vi "test-SwerveModuleState.vi"(8 "error in (no error)":errorcluster) -> (0 "error out":errorcluster, 3 "ALL TESTS PASSED":bool)   [LabVIEW 2019]
uses:
  <vilib>/Rock Robotics/WPI/ThirdParty/JAS_Junk/TrajLib/TypeDef/SWERVE_DRIVE_MODULE_STATE.ctl
  <vilib>/Rock Robotics/WPI/ThirdParty/JAS_Junk/TrajLib/TypeDef/ROTATION2D.ctl
  <vilib>/Rock Robotics/WPI/ThirdParty/JAS_Junk/TrajLib/Rotation2d_Minus.vi
  <vilib>/Rock Robotics/WPI/ThirdParty/JAS_Junk/TrajLib/Rotation2d_GetRadians.vi
  <vilib>/Rock Robotics/WPI/ThirdParty/JAS_Junk/TrajLib/Rotation2d_RotateBy.vi
  <vilib>/Rock Robotics/WPI/ThirdParty/JAS_Junk/TrajLib/Rotation2d_UnaryMinus.vi
  <vilib>/Rock Robotics/WPI/ThirdParty/JAS_Junk/TrajLib/Rotation2d_CreateXY.vi
  <vilib>/Rock Robotics/WPI/ThirdParty/JAS_Junk/TrajLib/Util_CalcDist.vi
  <vilib>/Rock Robotics/WPI/ThirdParty/JAS_Junk/TrajLib/Trajectory_Library.lvlib
panel:
  out "Test 4":bool
  out "Test 3":bool
  out "Test 1B":bool
  out "T1B":T1={"Speed"=0.0, "Angle"={"VALUE"=0.0, "COS"=1.0, "SIN"=0.0}} {"Angle"."SIN" format="%13.4f"; "Angle"."COS" format="%13.4f"; "Angle"."VALUE" format="%13.4f"}
  out "Test 1A":bool
  out "T1A":T1={"Speed"=0.0, "Angle"={"VALUE"=0.0, "COS"=1.0, "SIN"=0.0}} {"Angle"."SIN" format="%13.4f"; "Angle"."COS" format="%13.4f"; "Angle"."VALUE" format="%13.4f"}
  out "Test 0B":bool
  out "T0B":T1={"Speed"=0.0, "Angle"={"VALUE"=0.0, "COS"=1.0, "SIN"=0.0}} {"Angle"."SIN" format="%13.4f"; "Angle"."COS" format="%13.4f"; "Angle"."VALUE" format="%13.4f"}
  out "Test 0A":bool
  out "T91 Ang = reversed":T1={"Speed"=0.0, "Angle"={"VALUE"=0.0, "COS"=1.0, "SIN"=0.0}} {"Angle"."SIN" format="%13.4f"; "Angle"."COS" format="%13.4f"; "Angle"."VALUE" format="%13.4f"}
  out "T90  Ang = small":T1={"Speed"=0.0, "Angle"={"VALUE"=0.0, "COS"=1.0, "SIN"=0.0}} {"Angle"."SIN" format="%13.4f"; "Angle"."COS" format="%13.4f"; "Angle"."VALUE" format="%13.4f"}
  out "T3":T1={"Speed"=0.0, "Angle"={"VALUE"=0.0, "COS"=1.0, "SIN"=0.0}} {"Angle"."SIN" format="%13.4f"; "Angle"."COS" format="%13.4f"; "Angle"."VALUE" format="%13.4f"}
  out "T2":T1={"Speed"=0.0, "Angle"={"VALUE"=0.0, "COS"=1.0, "SIN"=0.0}} {"Angle"."SIN" format="%13.4f"; "Angle"."COS" format="%13.4f"; "Angle"."VALUE" format="%13.4f"}
  out "T1":i32
  out "T0A":T1={"Speed"=0.0, "Angle"={"VALUE"=0.0, "COS"=1.0, "SIN"=0.0}} {"Angle"."SIN" format="%13.4f"; "Angle"."COS" format="%13.4f"; "Angle"."VALUE" format="%13.4f"}
  # "SwerveModuleState Test"
  # "THESE ARE OLD TESTS..."
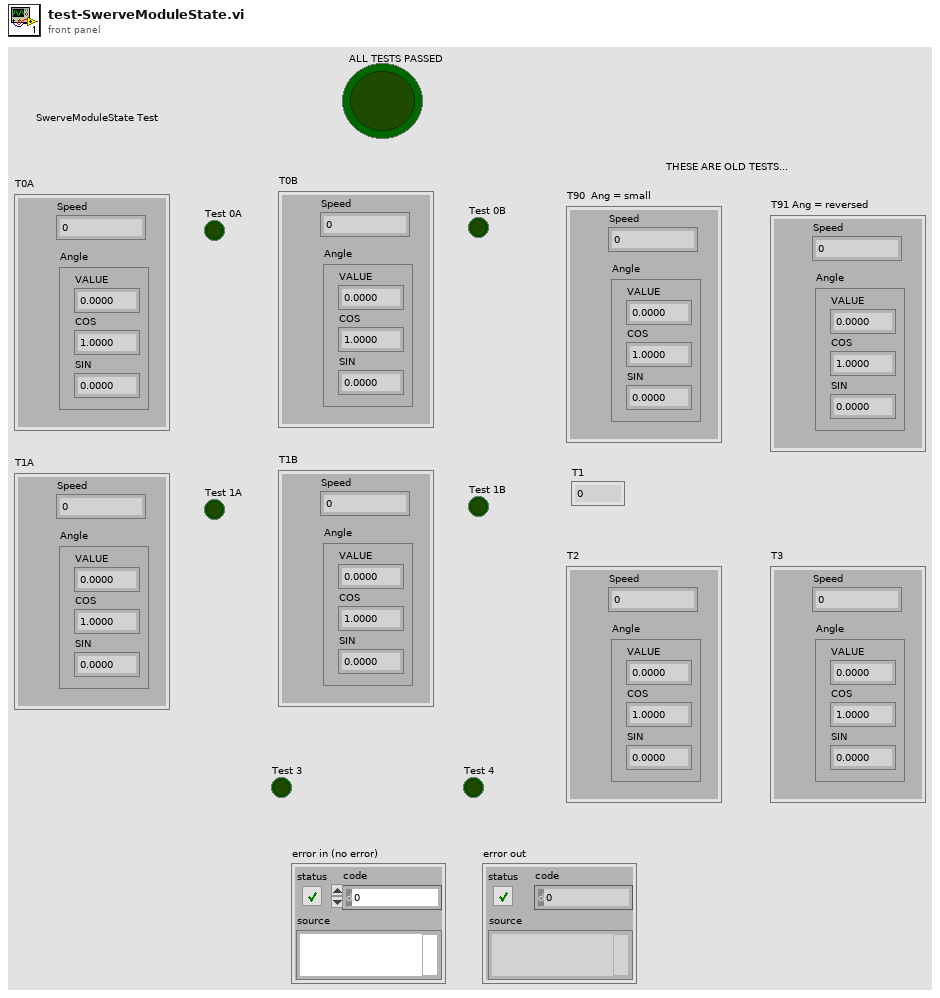
[diagram p1: front panel]
types:
  T1 = typedef "Trajectory_Library.lvlib/SWERVE_DRIVE_MODULE_STATE.ctl" = cluster{"Speed":dbl, "Angle":T2}
  T2 = typedef "Trajectory_Library.lvlib/ROTATION2D.ctl" = cluster{"VALUE":dbl, "COS":dbl, "SIN":dbl}
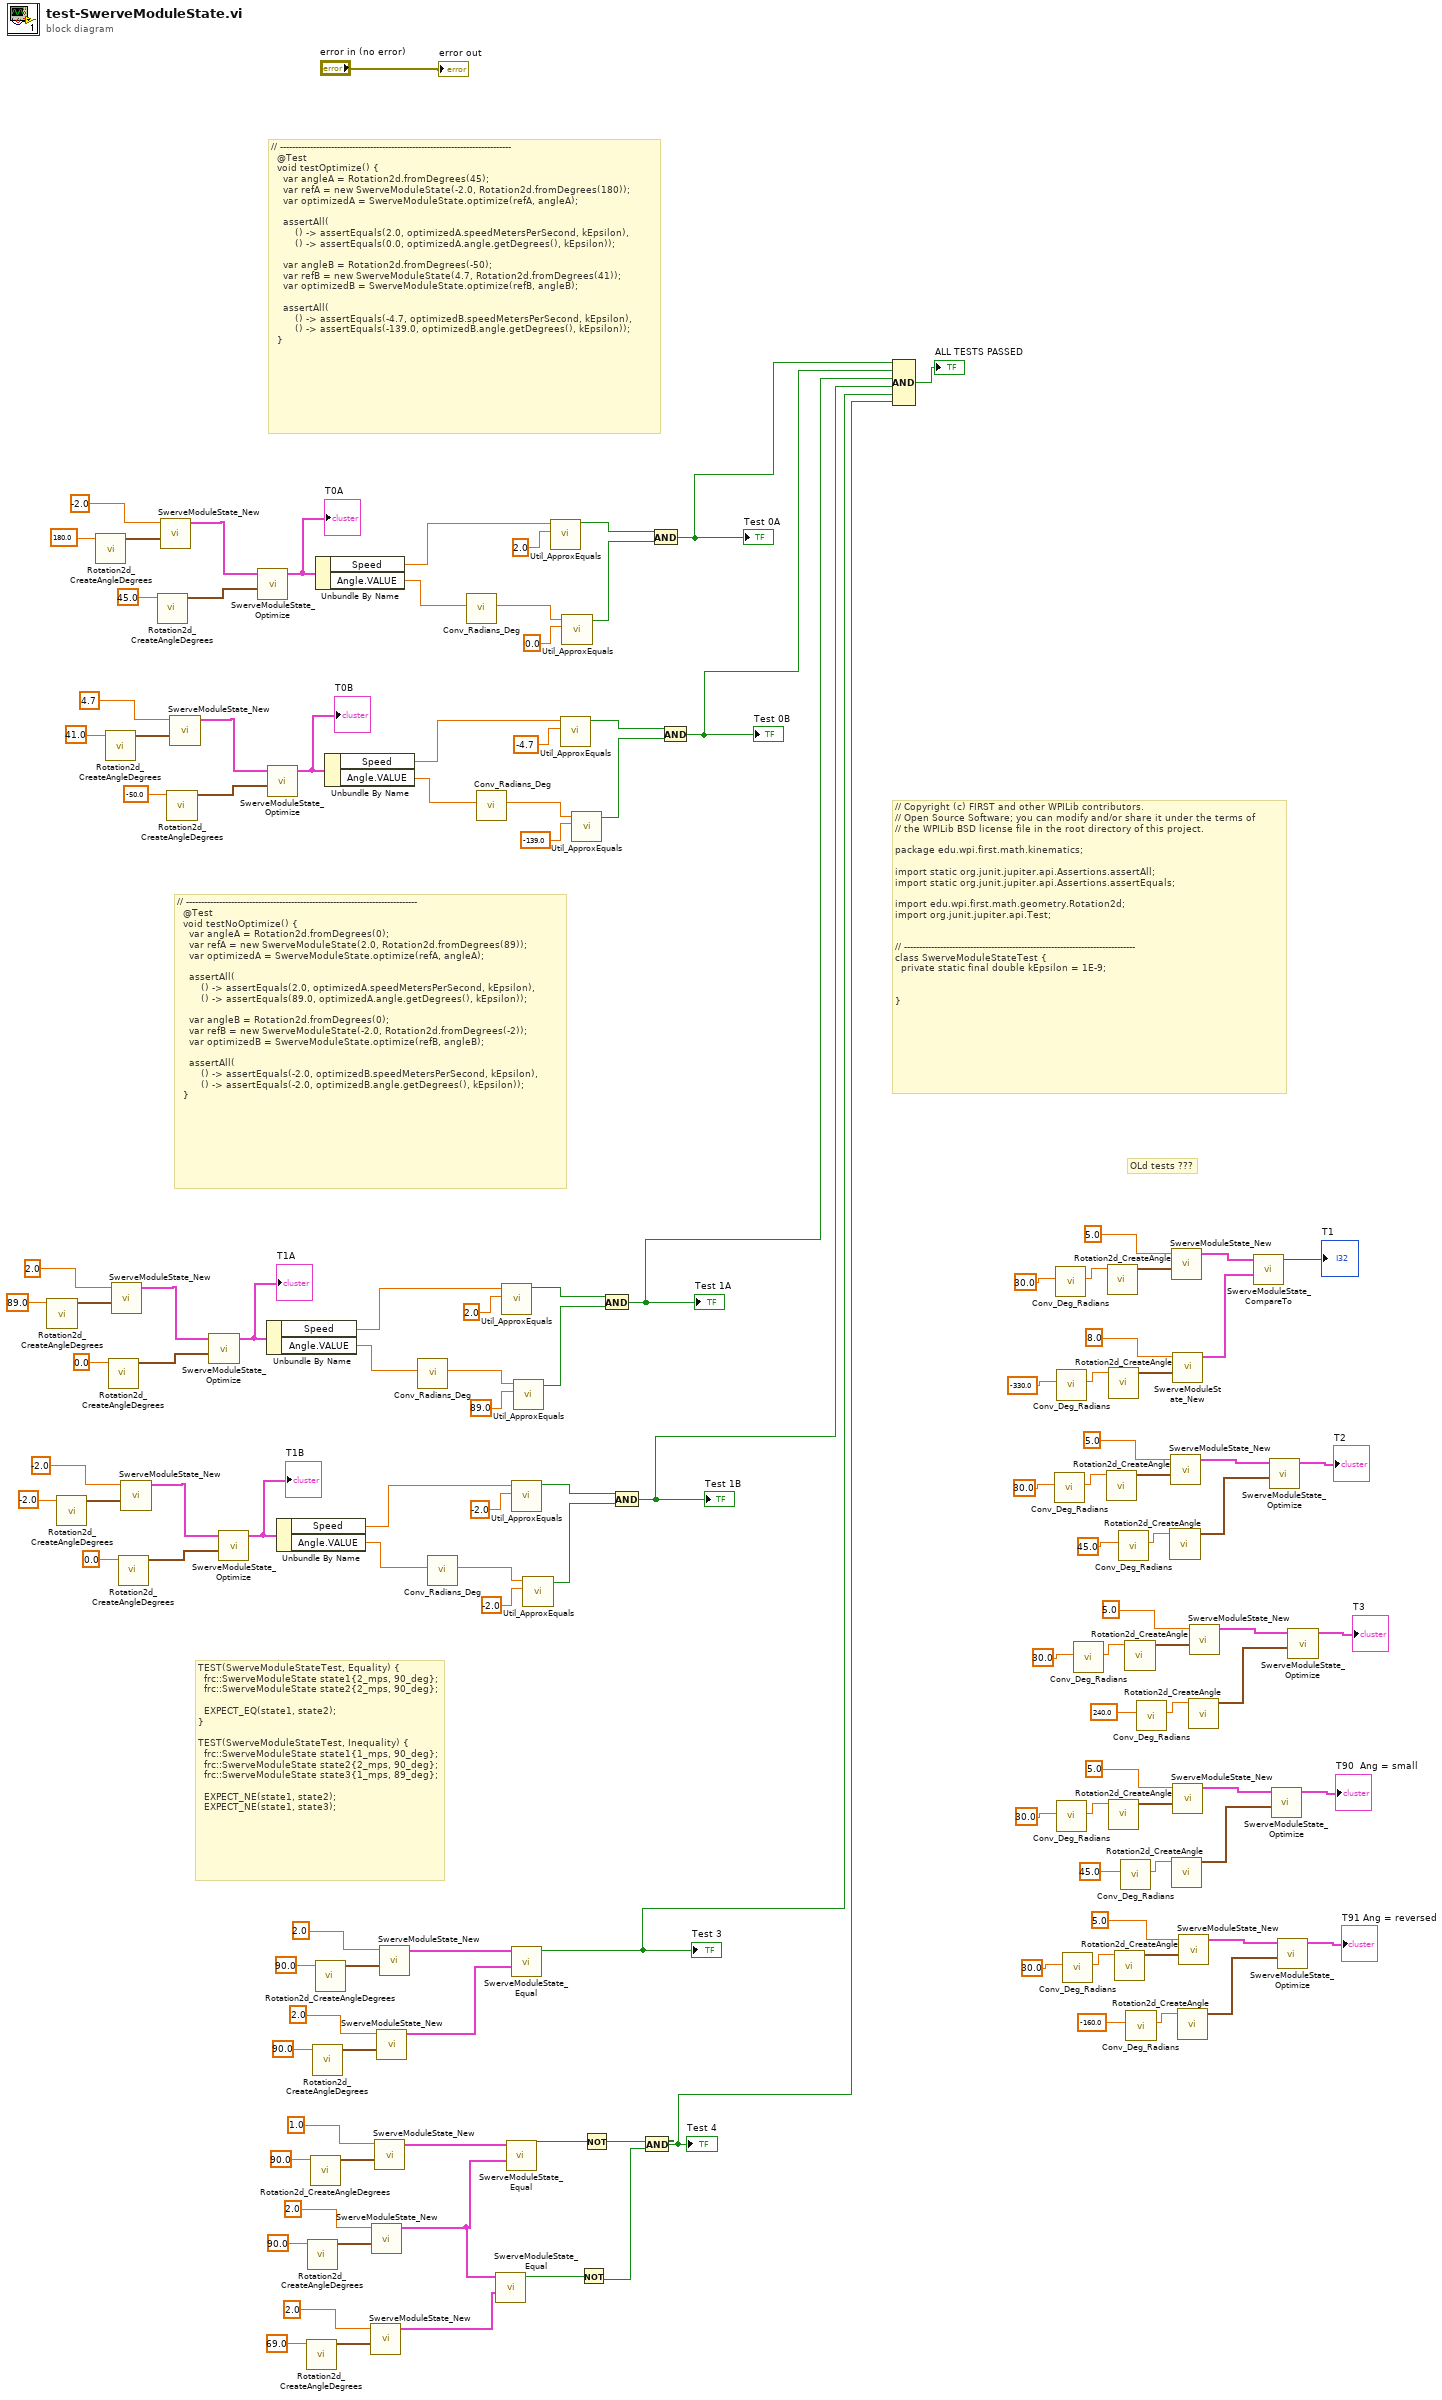
[diagram p0: block diagram]
diagram:
  # "TEST(SwerveModuleStateTest, Equality) {\n  frc::SwerveModuleState state1{2_mps, 90_deg};\n  frc::SwerveModuleState state2{2_mps, 90_deg};\n\n  EXPECT_EQ(state1, state2);\n}\n\nTEST(SwerveModuleStateTest, Inequality) {\n  frc::SwerveModuleState state1{1_mps, 90_deg};\n  frc::SwerveModuleState state2{2_mps, 90_deg};\n  frc::SwerveModuleState state3{1_mps, 89_deg};\n\n  EXPECT_NE(state1, state2);\n  EXPECT_NE(state1, state3);"
  # "OLd tests ???"
  # "// -----------------------------------------------------------------------------\n  @Test\n  void testNoOptimize() {\n    var angleA = Rotation2d.fromDegrees(0);\n    var refA = new SwerveModuleState(2.0, Rotation2d.fromDegrees(89));\n    var optimizedA = SwerveModuleState.optimize(refA, angleA);\n\n    assertAll(\n        () -> assertEquals(2.0, optimizedA.speedMetersPerSecond, kEpsilon),\n        () -> assertEquals(89.0, optimizedA.angle.getDegrees(), kEpsilon));\n\n    var angleB = Rotation2d.fromDegrees(0);\n    var refB = new SwerveModuleState(-2.0, Rotation2d.fromDegrees(-2));\n    var optimizedB = SwerveModuleState.optimize(refB, angleB);\n\n    assertAll(\n        () -> assertEquals(-2.0, optimizedB.speedMetersPerSecond, kEpsilon),\n        () -> assertEquals(-2.0, optimizedB.angle.getDegrees(), kEpsilon));\n  }"
  # "// -----------------------------------------------------------------------------\n  @Test\n  void testOptimize() {\n    var angleA = Rotation2d.fromDegrees(45);\n    var refA = new SwerveModuleState(-2.0, Rotation2d.fromDegrees(180));\n    var optimizedA = SwerveModuleState.optimize(refA, angleA);\n\n    assertAll(\n        () -> assertEquals(2.0, optimizedA.speedMetersPerSecond, kEpsilon),\n        () -> assertEquals(0.0, optimizedA.angle.getDegrees(), kEpsilon));\n\n    var angleB = Rotation2d.fromDegrees(-50);\n    var refB = new SwerveModuleState(4.7, Rotation2d.fromDegrees(41));\n    var optimizedB = SwerveModuleState.optimize(refB, angleB);\n\n    assertAll(\n        () -> assertEquals(-4.7, optimizedB.speedMetersPerSecond, kEpsilon),\n        () -> assertEquals(-139.0, optimizedB.angle.getDegrees(), kEpsilon));\n  }"
  # "// Copyright (c) FIRST and other WPILib contributors.\n// Open Source Software; you can modify and/or share it under the terms of\n// the WPILib BSD license file in the root directory of this project.\n\npackage edu.wpi.first.math.kinematics;\n\nimport static org.junit.jupiter.api.Assertions.assertAll;\nimport static org.junit.jupiter.api.Assertions.assertEquals;\n\nimport edu.wpi.first.math.geometry.Rotation2d;\nimport org.junit.jupiter.api.Test;\n\n\n// -----------------------------------------------------------------------------\nclass SwerveModuleStateTest {\n  private static final double kEpsilon = 1E-9;\n\n\n}"
  n1 = call <vilib>:"Rotation2d_CreateAngleDegrees.vi"("Angle_Degrees"=89.0 ("y")) -> ("ROTATION"=w56:T2)  [unwired: 10 in]
  n2 = call <vilib>:"Rotation2d_CreateAngleDegrees.vi"("Angle_Degrees"=-2.0 ("y")) -> ("ROTATION"=w42:T2)  [unwired: 10 in]
  n3 = call <vilib>:"Rotation2d_CreateAngleDegrees.vi"("Angle_Degrees"=180.0 ("y")) -> ("ROTATION"=w134:T2)  [unwired: 10 in]
  n4 = call <vilib>:"Rotation2d_CreateAngleDegrees.vi"("Angle_Degrees"=41.0 ("y")) -> ("ROTATION"=w72:T2)  [unwired: 10 in]
  n5 = call <vilib>:"Rotation2d_CreateAngleDegrees.vi"("Angle_Degrees"=0.0 ("y")) -> ("ROTATION"=w52:T2)  [unwired: 10 in]
  n6 = call <vilib>:"SwerveModuleState_New.vi"("ROTATION"=w56, "Speed"=2.0) -> ("SWERVE_DRIVE_MODULE_STATE"=w53:T1)  [unwired: 9 in]
  n7 = call <vilib>:"Rotation2d_CreateAngleDegrees.vi"("Angle_Degrees"=0.0 ("y")) -> ("ROTATION"=w38:T2)  [unwired: 10 in]
  n8 = call <vilib>:"SwerveModuleState_New.vi"("ROTATION"=w42, "Speed"=-2.0) -> ("SWERVE_DRIVE_MODULE_STATE"=w39:T1)  [unwired: 9 in]
  n9 = call <vilib>:"Rotation2d_CreateAngleDegrees.vi"("Angle_Degrees"=45.0 ("y")) -> ("ROTATION"=w83:T2)  [unwired: 10 in]
  n10 = call <vilib>:"SwerveModuleState_New.vi"("ROTATION"=w134, "Speed"=-2.0) -> ("SWERVE_DRIVE_MODULE_STATE"=w84:T1)  [unwired: 9 in]
  n11 = call <vilib>:"Rotation2d_CreateAngleDegrees.vi"("Angle_Degrees"=-50.0 ("y")) -> ("ROTATION"=w68:T2)  [unwired: 10 in]
  n12 = call <vilib>:"SwerveModuleState_New.vi"("ROTATION"=w72, "Speed"=4.7) -> ("SWERVE_DRIVE_MODULE_STATE"=w69:T1)  [unwired: 9 in]
  n13 = call <vilib>:"SwerveModuleState_Optimize.vi"("CurrentAngle"=w52, "Desired State"=w53) -> ("out SWERVE_DRIVE_MODULE_STATE"=w46:T1)  [unwired: 9 in]
  "T1A" <- w46
  n14 = call <vilib>:"SwerveModuleState_Optimize.vi"("CurrentAngle"=w38, "Desired State"=w39) -> ("out SWERVE_DRIVE_MODULE_STATE"=w32:T1)  [unwired: 9 in]
  "T1B" <- w32
  n15 = call <vilib>:"SwerveModuleState_Optimize.vi"("CurrentAngle"=w83, "Desired State"=w84) -> ("out SWERVE_DRIVE_MODULE_STATE"=w77:T1)  [unwired: 9 in]
  "T0A" <- w77
  n16 = Unbundle By Name(w46) -> ("Speed"=w47:dbl, "Angle.VALUE"=w51:dbl)
  n17 = call <vilib>:"SwerveModuleState_Optimize.vi"("CurrentAngle"=w68, "Desired State"=w69) -> ("out SWERVE_DRIVE_MODULE_STATE"=w62:T1)  [unwired: 9 in]
  "T0B" <- w62
  n18 = Unbundle By Name(w32) -> ("Speed"=w33:dbl, "Angle.VALUE"=w37:dbl)
  n19 = call <vilib>:"Rotation2d_CreateAngleDegrees.vi"("Angle_Degrees"=69.0 ("y")) -> ("ROTATION"=w10:T2)  [unwired: 10 in]
  n20 = call <vilib>:"Rotation2d_CreateAngleDegrees.vi"("Angle_Degrees"=90.0 ("y")) -> ("ROTATION"=w14:T2)  [unwired: 10 in]
  n21 = call <vilib>:"Rotation2d_CreateAngleDegrees.vi"("Angle_Degrees"=90.0 ("y")) -> ("ROTATION"=w17:T2)  [unwired: 10 in]
  n22 = call <vilib>:"Rotation2d_CreateAngleDegrees.vi"("Angle_Degrees"=90.0 ("y")) -> ("ROTATION"=w22:T2)  [unwired: 10 in]
  n23 = Unbundle By Name(w77) -> ("Speed"=w78:dbl, "Angle.VALUE"=w82:dbl)
  n24 = call <vilib>:"Rotation2d_CreateAngleDegrees.vi"("Angle_Degrees"=90.0 ("y")) -> ("ROTATION"=w25:T2)  [unwired: 10 in]
  n25 = Unbundle By Name(w62) -> ("Speed"=w63:dbl, "Angle.VALUE"=w67:dbl)
  n26 = call <vilib>:"SwerveModuleState_New.vi"("ROTATION"=w10, "Speed"=2.0) -> ("SWERVE_DRIVE_MODULE_STATE"=w7:T1)  [unwired: 9 in]
  n27 = call <vilib>:"SwerveModuleState_New.vi"("ROTATION"=w14, "Speed"=2.0) -> ("SWERVE_DRIVE_MODULE_STATE"=w8:T1)  [unwired: 9 in]
  n28 = call <vilib>:"SwerveModuleState_New.vi"("ROTATION"=w17, "Speed"=1.0) -> ("SWERVE_DRIVE_MODULE_STATE"=w12:T1)  [unwired: 9 in]
  n29 = call <vilib>:"SwerveModuleState_New.vi"("ROTATION"=w22, "Speed"=2.0) -> ("SWERVE_DRIVE_MODULE_STATE"=w19:T1)  [unwired: 9 in]
  n30 = call <vilib>:"SwerveModuleState_New.vi"("ROTATION"=w25, "Speed"=2.0) -> ("SWERVE_DRIVE_MODULE_STATE"=w20:T1)  [unwired: 9 in]
  n31 = call <vilib>:"Conv_Radians_Deg.vi"("Radians"=w51) -> ("Degrees"=w48:dbl)  [unwired: 10 in]
  n32 = call <vilib>:"Conv_Radians_Deg.vi"("Radians"=w37) -> ("Degrees"=w34:dbl)  [unwired: 10 in]
  n33 = call <vilib>:"Conv_Radians_Deg.vi"("Radians"=w82) -> ("Degrees"=w79:dbl)  [unwired: 10 in]
  n34 = call <vilib>:"Conv_Radians_Deg.vi"("Radians"=w67) -> ("Degrees"=w64:dbl)  [unwired: 10 in]
  n35 = call <vilib>:"SwerveModuleState_Equal.vi"("other SWERVE_DRIVE_MODULE_STATE"=w7, "in SWERVE_DRIVE_MODULE_STATE"=w8) -> ("Equal"=w6:bool)  [unwired: 9 in]
  n36 = call <vilib>:"Util_ApproxEquals.vi"("Value 2"=2.0, "Value 1"=w47) -> ("ApproxEquals"=w45:bool)  [unwired: 9 in]
  n37 = call <vilib>:"SwerveModuleState_Equal.vi"("other SWERVE_DRIVE_MODULE_STATE"=w8, "in SWERVE_DRIVE_MODULE_STATE"=w12) -> ("Equal"=w5:bool)  [unwired: 9 in]
  n38 = call <vilib>:"Util_ApproxEquals.vi"("Value 2"=-2.0, "Value 1"=w33) -> ("ApproxEquals"=w31:bool)  [unwired: 9 in]
  n39 = call <vilib>:"SwerveModuleState_Equal.vi"("other SWERVE_DRIVE_MODULE_STATE"=w19, "in SWERVE_DRIVE_MODULE_STATE"=w20) -> ("Equal"=w2:bool)  [unwired: 9 in]
  "Test 3" <- w2
  n40 = call <vilib>:"Util_ApproxEquals.vi"("Value 2"=89.0, "Value 1"=w48) -> ("ApproxEquals"=w44:bool)  [unwired: 9 in]
  n41 = call <vilib>:"Util_ApproxEquals.vi"("Value 2"=-2.0, "Value 1"=w34) -> ("ApproxEquals"=w30:bool)  [unwired: 9 in]
  n42 = call <vilib>:"Util_ApproxEquals.vi"("Value 2"=2.0, "Value 1"=w78) -> ("ApproxEquals"=w76:bool)  [unwired: 9 in]
  n43 = call <vilib>:"Util_ApproxEquals.vi"("Value 2"=-4.7, "Value 1"=w63) -> ("ApproxEquals"=w61:bool)  [unwired: 9 in]
  n44 = call <vilib>:"Util_ApproxEquals.vi"("Value 2"=0.0, "Value 1"=w79) -> ("ApproxEquals"=w75:bool)  [unwired: 9 in]
  n45 = call <vilib>:"Util_ApproxEquals.vi"("Value 2"=-139.0, "Value 1"=w64) -> ("ApproxEquals"=w60:bool)  [unwired: 9 in]
  n46 = Not(x=w6) -> (.not. x?=w3:bool)
  n47 = Not(x=w5) -> (.not. x?=w4:bool)
  n48 = And(x=w45, y=w44) -> (x .and. y?=w29:bool)
  "Test 1A" <- w29
  n49 = And(x=w31, y=w30) -> (x .and. y?=w28:bool)
  "Test 1B" <- w28
  n50 = And(x=w4, y=w3) -> (x .and. y?=w1:bool)
  "Test 4" <- w1
  n51 = And(x=w76, y=w75) -> (x .and. y?=w74:bool)
  "Test 0A" <- w74
  n52 = And(x=w61, y=w60) -> (x .and. y?=w59:bool)
  "Test 0B" <- w59
  n53 = Compound Arithmetic op=AND(w74, w59, w29, w28, w2, w1) -> (→"ALL TESTS PASSED":bool)
  n54 = call <vilib>:"Conv_Deg_Radians.vi"("Degress"=30.0 ("y")) -> ("Radians"=w122:dbl)  [unwired: 10 in]
  n55 = call <vilib>:"Conv_Deg_Radians.vi"("Degress"=30.0 ("y")) -> ("Radians"=w133:dbl)  [unwired: 10 in]
  n56 = call <vilib>:"Conv_Deg_Radians.vi"("Degress"=-330.0 ("y")) -> ("Radians"=w129:dbl)  [unwired: 10 in]
  n57 = call <vilib>:"Conv_Deg_Radians.vi"("Degress"=30.0 ("y")) -> ("Radians"=w104:dbl)  [unwired: 10 in]
  n58 = call <vilib>:"Conv_Deg_Radians.vi"("Degress"=30.0 ("y")) -> ("Radians"=w95:dbl)  [unwired: 10 in]
  n59 = call <vilib>:"Conv_Deg_Radians.vi"("Degress"=30.0 ("y")) -> ("Radians"=w113:dbl)  [unwired: 10 in]
  n60 = call <vilib>:"Rotation2d_CreateAngle.vi"("Angle"=w122) -> ("ROTATION"=w119:T2)  [unwired: 10 in]
  n61 = call <vilib>:"Rotation2d_CreateAngle.vi"("Angle"=w133) -> ("ROTATION"=w130:T2)  [unwired: 10 in]
  n62 = call <vilib>:"Rotation2d_CreateAngle.vi"("Angle"=w129) -> ("ROTATION"=w126:T2)  [unwired: 10 in]
  n63 = call <vilib>:"Rotation2d_CreateAngle.vi"("Angle"=w104) -> ("ROTATION"=w102:T2)  [unwired: 10 in]
  n64 = call <vilib>:"Rotation2d_CreateAngle.vi"("Angle"=w95) -> ("ROTATION"=w93:T2)  [unwired: 10 in]
  n65 = call <vilib>:"Conv_Deg_Radians.vi"("Degress"=45.0 ("y")) -> ("Radians"=w116:dbl)  [unwired: 10 in]
  n66 = call <vilib>:"Conv_Deg_Radians.vi"("Degress"=45.0 ("y")) -> ("Radians"=w99:dbl)  [unwired: 10 in]
  n67 = call <vilib>:"Rotation2d_CreateAngle.vi"("Angle"=w113) -> ("ROTATION"=w111:T2)  [unwired: 10 in]
  n68 = call <vilib>:"Conv_Deg_Radians.vi"("Degress"=-160.0 ("y")) -> ("Radians"=w90:dbl)  [unwired: 10 in]
  n69 = call <vilib>:"Conv_Deg_Radians.vi"("Degress"=240.0 ("y")) -> ("Radians"=w108:dbl)  [unwired: 10 in]
  n70 = call <vilib>:"Rotation2d_CreateAngle.vi"("Angle"=w116) -> ("ROTATION"=w114:T2)  [unwired: 10 in]
  n71 = call <vilib>:"SwerveModuleState_New.vi"("ROTATION"=w119, "Speed"=5.0) -> ("SWERVE_DRIVE_MODULE_STATE"=w118:T1)  [unwired: 9 in]
  n72 = call <vilib>:"SwerveModuleState_New.vi"("ROTATION"=w130, "Speed"=5.0) -> ("SWERVE_DRIVE_MODULE_STATE"=w124:T1)  [unwired: 9 in]
  n73 = call <vilib>:"Rotation2d_CreateAngle.vi"("Angle"=w99) -> ("ROTATION"=w97:T2)  [unwired: 10 in]
  n74 = call <vilib>:"SwerveModuleState_New.vi"("ROTATION"=w126, "Speed"=8.0) -> ("SWERVE_DRIVE_MODULE_STATE"=w123:T1)  [unwired: 9 in]
  n75 = call <vilib>:"SwerveModuleState_New.vi"("ROTATION"=w102, "Speed"=5.0) -> ("SWERVE_DRIVE_MODULE_STATE"=w101:T1)  [unwired: 9 in]
  n76 = call <vilib>:"Rotation2d_CreateAngle.vi"("Angle"=w90) -> ("ROTATION"=w88:T2)  [unwired: 10 in]
  n77 = call <vilib>:"SwerveModuleState_New.vi"("ROTATION"=w93, "Speed"=5.0) -> ("SWERVE_DRIVE_MODULE_STATE"=w92:T1)  [unwired: 9 in]
  n78 = call <vilib>:"Rotation2d_CreateAngle.vi"("Angle"=w108) -> ("ROTATION"=w106:T2)  [unwired: 10 in]
  n79 = call <vilib>:"SwerveModuleState_New.vi"("ROTATION"=w111, "Speed"=5.0) -> ("SWERVE_DRIVE_MODULE_STATE"=w110:T1)  [unwired: 9 in]
  n80 = call <vilib>:"SwerveModuleState_CompareTo.vi"("other SWERVE_DRIVE_MODULE_STATE"=w123, "in SWERVE_DRIVE_MODULE_STATE"=w124) -> ("Compare"=→"T1":i32)  [unwired: 9 in]
  n81 = call <vilib>:"SwerveModuleState_Optimize.vi"("CurrentAngle"=w114, "Desired State"=w118) -> ("out SWERVE_DRIVE_MODULE_STATE"=→"T2":T1)  [unwired: 9 in]
  n82 = call <vilib>:"SwerveModuleState_Optimize.vi"("CurrentAngle"=w97, "Desired State"=w101) -> ("out SWERVE_DRIVE_MODULE_STATE"=→"T90  Ang = small":T1)  [unwired: 9 in]
  n83 = call <vilib>:"SwerveModuleState_Optimize.vi"("CurrentAngle"=w88, "Desired State"=w92) -> ("out SWERVE_DRIVE_MODULE_STATE"=→"T91 Ang = reversed":T1)  [unwired: 9 in]
  n84 = call <vilib>:"SwerveModuleState_Optimize.vi"("CurrentAngle"=w106, "Desired State"=w110) -> ("out SWERVE_DRIVE_MODULE_STATE"=→"T3":T1)  [unwired: 9 in]
  "error out" <- "error in (no error)"
